vi "SetI2C.vi"(8 "error in (no error)":errorcluster, 9 "I2C Slave Address":u8=4, 10 "I2C":refnum<class "I2C.lvclass">, 11 "GrovePi in":refnum<class "GrovePi.lvclass">) -> (0 "error out":errorcluster, 3 "GrovePi out":refnum<class "GrovePi.lvclass">)   [LabVIEW 2014, in "GrovePi.lvclass"]
doc: "Sets the I2C bus to use and the I2C Slave Address for communicating to the GrovePi."
uses:
  GrovePi.lvclass
  I2C/I2C.lvclass
  GrovePi.lvclass/GrovePi.ctl
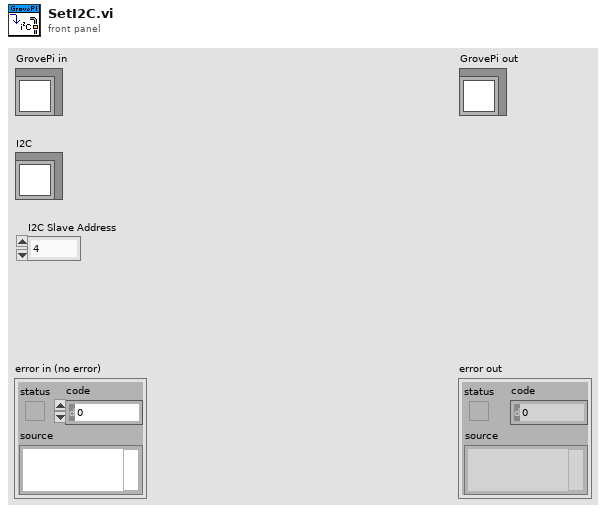
[diagram p1: front panel]
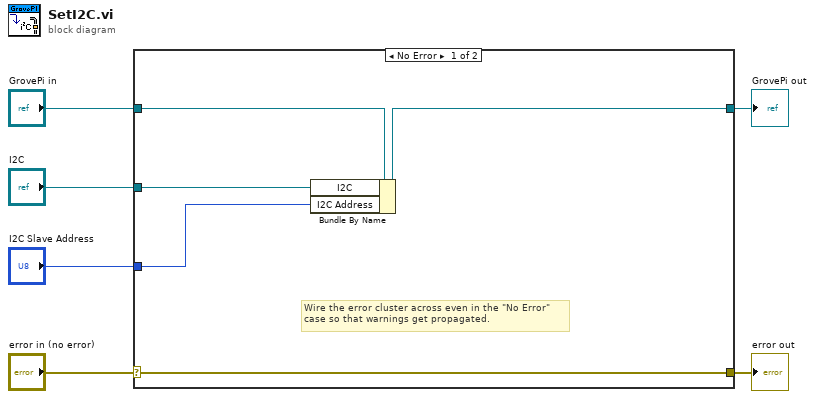
[diagram p0: block diagram]
diagram:
  n1 = case shown="No Error" "error in (no error)" {
    selector: "error in (no error)" -> [w10 w13]
    tunnel: [w10 w13] -> w5
    tunnel: [w9 w12] -> w3
    tunnel: "GrovePi in" -> [w11 w12]
    tunnel: "I2C" -> [w8 _]
    tunnel: "I2C Slave Address" -> [w7 _]
    frame No Error {
      # "Wire the error cluster across even in the \"No Error\"\ncase so that warnings get propagated."
      n2 = Bundle By Name(cluster=w11, "I2C"=w8, "I2C Address"=w7) -> (w9:refnum<class "GrovePi.lvclass">)
    }
    frame Error {
    }
  }
  "error out" <- w5
  "GrovePi out" <- w3
